vi "Read Hold plot upper.vi"(8 "error in (no error)":errorcluster, 11 "Scope5761":refnum<class "Scope5782_six_channel.lvclass">) -> (0 "error out":errorcluster, 2 "Hold plot upper":bool caption="Hold plot", 3 "Scope5761":refnum<class "Scope5782_six_channel.lvclass">)   [LabVIEW 2018, in "Scope5782_six_channel.lvclass"]
uses:
  Scope5782_six_channel.lvclass
  Scope5782_six_channel.lvclass/Scope5782_six_channel.ctl
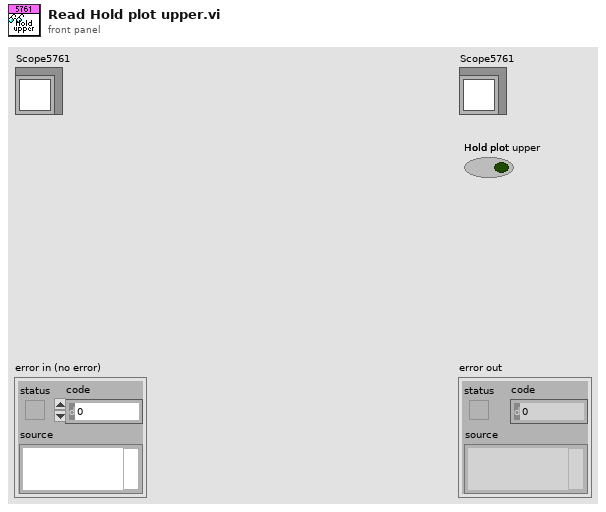
[diagram p1: front panel]
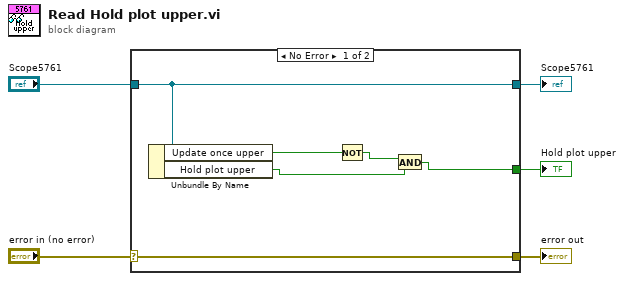
[diagram p0: block diagram]
diagram:
  n1 = case shown="No Error" "error in (no error)" {
    selector: "error in (no error)" -> [w11 w12]
    tunnel: [w11 w12] -> w4
    tunnel: [w10 w13] -> w2
    tunnel: "Scope5761" -> [w10 w13]
    tunnel: [w6 _] -> w1
    frame No Error {
      n2 = Unbundle By Name(w10) -> ("Update once upper"=w8:bool, "Hold plot upper"=w7:bool)
      n3 = Not(x=w8) -> (.not. x?=w9:bool)
      n4 = And(x=w9, y=w7) -> (x .and. y?=w6:bool)
    }
    frame Error {
    }
  }
  "error out" <- w4
  "Scope5761" <- w2
  "Hold plot upper" <- w1
